vi "Image to luminosity gradient complex map.vi"(2 "Error In":errorcluster, 3 "ROI to crop (pixels)":T1={"Xmax"=2147483647, "Ymax"=2147483647, "Xmin"=0, "Ymin"=0}, 4 "Image":T2) -> (0 "Error Out":errorcluster, 1 "Luminosity gradient map (complex)":cdb[][](array[numeric]))   [LabVIEW 2014]
uses:
  <vilib>/vision/Image Controls.llb/IMAQ Image.ctl
  Typedefs/ROI bounds.ctl
  <vilib>/Analysis/2dsp.llb/2D Convolution (DBL).vi
  <vilib>/vision/NI_Vision_Development_Module.lvlib
  <vilib>/Analysis/NI_AALPro.lvlib
panel:
  # "Paul Nathan 03/06/2015, 18/06/2015"
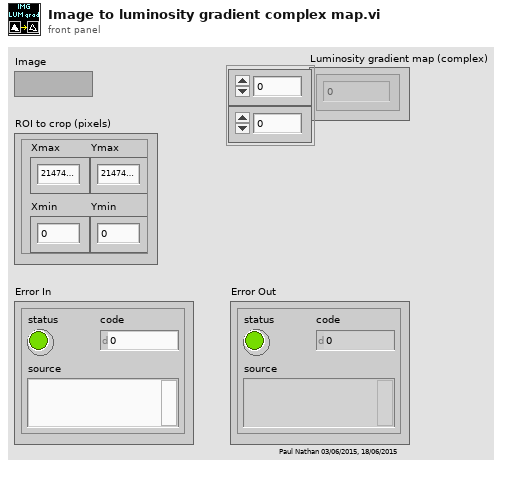
[diagram p1: front panel]
types:
  T1 = typedef "ROI bounds.ctl" = cluster{"Xmax":i32, "Ymax":i32, "Xmin":i32, "Ymin":i32}
  T2 = typedef "IMAQ Image.ctl" = refnum<image>
  T3 = cluster{"Red (or Hue) value":u8, "Green (or Sat) value":u8, "Blue (or Light or Val) value":u8}[][]
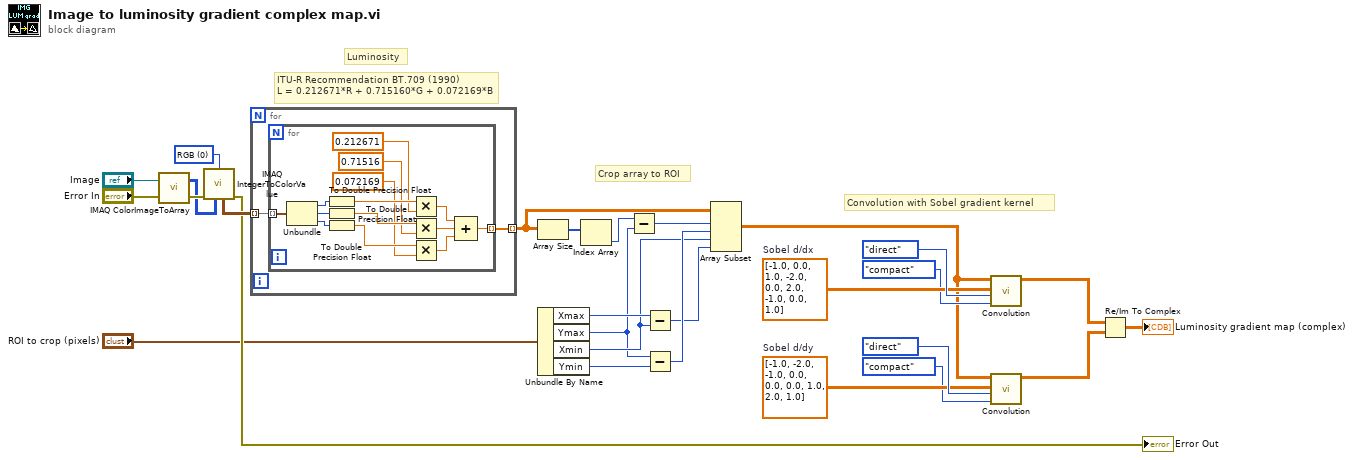
[diagram p0: block diagram]
diagram:
  w20 = dbl[][] [[-1.0, -2.0, -1.0], [0.0, 0.0, 0.0], [1.0, 2.0, 1.0]]  # Sobel d/dy
  w23 = dbl[][] [[-1.0, 0.0, 1.0], [-2.0, 0.0, 2.0], [-1.0, 0.0, 1.0]]  # Sobel d/dx
  w25 = u16 0 items=["RGB", "HSL", "HSV", "HSI"] ("Color Mode")
  # "Crop array to ROI"
  # "Convolution with Sobel gradient kernel"
  # "Luminosity"
  # "ITU-R Recommendation BT.709 (1990)\nL = 0.212671*R + 0.715160*G + 0.072169*B"
  n1 = call "IMAQ ColorImageToArray"("Image"="Image", "error in (no error)"="Error In") -> ("Image Pixels (U32)"=w26:u32[][], "error out"=w28:errorcluster)  [unwired: 2 in, 1 out]
  n2 = call "IMAQ IntegerToColorValue"("error in (no error)"=w28, "2D U32 array"=w26, "Color Mode"=w25) -> ("2D Color value array"=w27:T3, "error out"=→"Error Out":errorcluster)  [unwired: 2 in, 2 out]
  n3 = for {
    tunnel: w27 -> [w30] mode=indexing
    tunnel: [w29] -> w11 mode=indexing
    n4 = for {
      tunnel: w30 -> [w44] mode=indexing
      tunnel: [w31] -> w29 mode=indexing
      n5 = Unbundle(w44) -> ("Red (or Hue) value"=w43:u8, "Green (or Sat) value"=w41:u8, "Blue (or Light or Val) value"=w42:u8)
      n6 = To Double Precision Float(number=w43) -> (double precision float=w40:dbl)
      n7 = To Double Precision Float(number=w41) -> (double precision float=w39:dbl)
      n8 = To Double Precision Float(number=w42) -> (double precision float=w38:dbl)
      n9 = Multiply(x=w40, y=0.212671) -> (x*y=w34:dbl)
      n10 = Multiply(x=w39, y=0.71516) -> (x*y=w33:dbl)
      n11 = Multiply(x=w38, y=0.072169) -> (x*y=w32:dbl)
      n12 = Compound Arithmetic op=ADD(w34, w33, w32) -> (w31:dbl)
    }
  }
  n13 = Array Size(array=w11) -> (size(s)=w5:i32[])
  n14 = Unbundle By Name("ROI to crop (pixels)") -> ("Xmax"=w9:i32, "Ymax"=w1:i32, "Xmin"=w6:i32, "Ymin"=w3:i32)
  n15 = Index Array(array=w5) -> (element=w4:i32)  [unwired: 1 in]
  n16 = Subtract(x=w4, y=w1) -> (x-y=w2:i32)
  n17 = Subtract(x=w9, y=w6) -> (x-y=w7:i32)
  n18 = Subtract(x=w1, y=w3) -> (x-y=w8:i32)
  n19 = Array Subset(array=w11, index (row)=w2, length (row)=w8, index (col)=w6, length (col)=w7) -> (w12:dbl[][])
  n20 = call-poly <vilib>:"Convolution.vi"("output size"=enum32{"full", "size X", "compact"}."compact", "algorithm"=enum32{"direct", "frequency domain"}."direct", "Y"=w23, "X"=w12) -> ("X * Y"=w19:dbl[][])  [unwired: 6 in, 1 out]
  n21 = call-poly <vilib>:"Convolution.vi"("output size"=enum32{"full", "size X", "compact"}."compact", "algorithm"=enum32{"direct", "frequency domain"}."direct", "Y"=w20, "X"=w12) -> ("X * Y"=w18:dbl[][])  [unwired: 6 in, 1 out]
  n22 = Re/Im To Complex(1:w18, 2:w19) -> (0:→"Luminosity gradient map (complex)":cdb[][])
